vi "IIR Filter for N Chan-modified.vi"(4 "optional IIR filter specifications":T2={"Lower PB"=100.0, "Upper PB"=0.0, "Lower SB"=200.0, "Upper SB"=0.0, "PB Gain"=0.0, "SB Gain"=-60.0, "Scale"=TRUE} {"PB Gain" format="%0.2f"; "SB Gain" format="%0.2f"; "Lower SB" format="%0.2p"; "Upper SB" format="%0.2f"; "Lower PB" format="%0.2p"; "Upper PB" format="%0.2f"}, 6 "IIR filter specifications":T3={"Topology"=enum."Butterworth", "Type"=enum."Lowpass", "Order"=1, "Lower Fc"=100.0, "Upper Fc"=200.0, "PB Ripple"=1.0, "SB Attenuation"=60.0} {"PB Ripple" format="%0.2f"; "Lower Fc" format="%0.2p"; "SB Attenuation" format="%0.2f"; "Upper Fc" format="%0.2p"}, 7 "reset filters":bool, 8 "error in (no error)":errorcluster, 11 "signal(s) in":waveform(dbl)[](array[waveform])) -> (0 "error out":errorcluster, 2 "filter information":T1 {"phase H(w)"."df" format="%.2p"; "phase H(w)"."f0" format="%.2p"; "phase H(w)"."Phase H(w)" format="%.2p"; "magnitude H(w)"."df" format="%.2p"; "magnitude H(w)"."f0" format="%.2p"; "magnitude H(w)"."Mag H(w)" format="%.2p"}, 3 "signal(s) out":waveform(dbl)[](array[waveform]))   [LabVIEW 2015]
doc: "Filters signals in either single or multiple waveforms. If you are filtering multiple waveforms, the VI maintains separate filter states for each waveform. The data types you wire to the <B>signal in</B> and <B>IIR filter specifications</B> inputs determine the polymorphic instance to use."
uses:
  <vilib>/measure/maUtilsandCtls.llb/ma_array_Check Time Signal Continuity.vi
  <vilib>/measure/NI_MAPro.lvlib
  <vilib>/measure/NI_MABase.lvlib
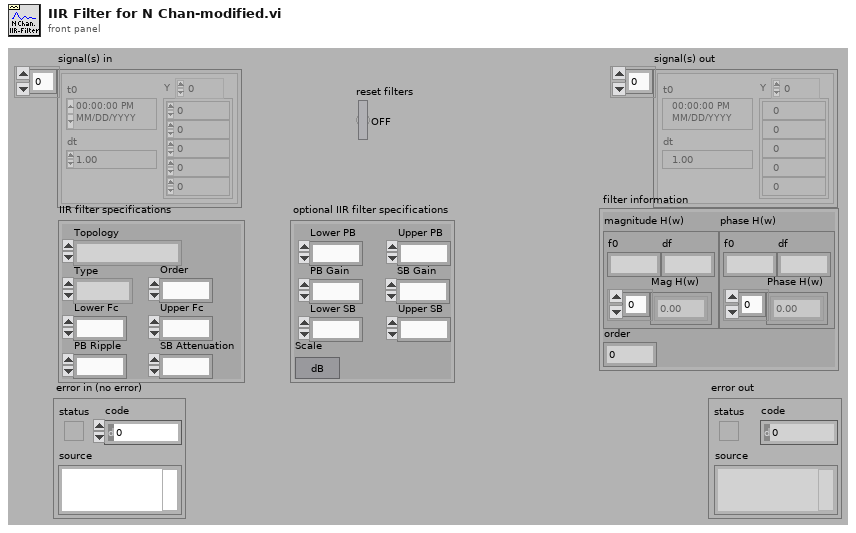
[diagram p1: front panel]
types:
  T1 = cluster{"magnitude H(w)":cluster{"f0":dbl, "df":dbl, "Mag H(w)":dbl[]}, "phase H(w)":cluster{"f0":dbl, "df":dbl, "Phase H(w)":dbl[]}, "order":i32}
  T2 = cluster{"Lower PB":dbl, "Upper PB":dbl, "Lower SB":dbl, "Upper SB":dbl, "PB Gain":dbl, "SB Gain":dbl, "Scale":bool}
  T3 = cluster{"Topology":enum16{"Off", "Butterworth", "Chebyshev", "Inverse Chebyshev", "Elliptic", "Bessel"}, "Type":enum16{"Lowpass", "Highpass", "Bandpass", "Bandstop"}, "Order":i32, "Lower Fc":dbl, "Upper Fc":dbl, "PB Ripple":dbl, "SB Attenuation":dbl}
  T4 = cluster{"filter structure":enum32{"IIR 2nd Order", "IIR 4th Order"}, "Reverse Coefficients":dbl[], "Forward Coefficients":dbl[]}
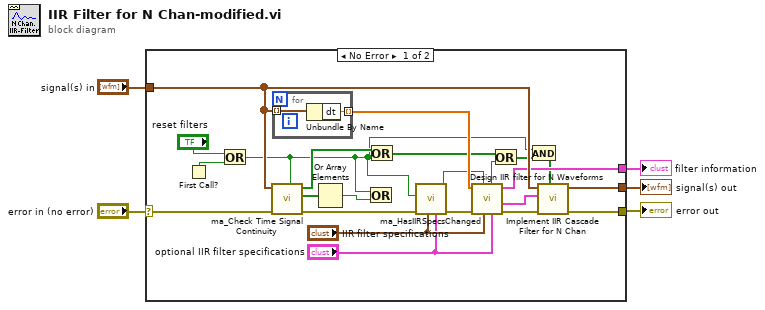
[diagram p0: block diagram]
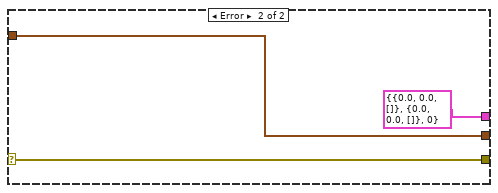
[diagram p2: hidden frame]
diagram:
  n1 = case shown="No Error" "error in (no error)" {
    selector: "error in (no error)" -> [w25 w32]
    tunnel: "signal(s) in" -> [w27 w33]
    tunnel: [w28 w32] -> w4
    tunnel: [w26 w33] -> w3
    tunnel: [w24 T1 {"magnitude H(w)"={"f0"=0.0, "df"=0.0, "Mag H(w)"=[]}, "phase H(w)"={"f0"=0.0, "df"=0.0, "Phase H(w)"=[]}, "order"=0} ("Filter Information")] -> w1
    frame No Error {
      n2 = First Call?() -> (First Call?: T/F=w10:bool)
      n3 = Or(x="reset filters", y=w10) -> (x .or. y?=w6:bool)
      n4 = call-poly <vilib>:"ma_Check Time Signal Continuity.vi"("Ignore input time stamp"=w6, "error in (no error)"=w25, "waveforms"=w27) -> ("error out"=w16:errorcluster, "dt changed"=w20:bool[], "t0 changed"=w13:bool[])  [unwired: 5 in, 1 out]
      n5 = for {
        tunnel: w27 -> [w30] mode=indexing
        tunnel: [w29] -> w21 mode=indexing
        n6 = Unbundle By Name(w30) -> ("dt"=w29:dbl)
      }
      n7 = Or Array Elements(Boolean array=w20) -> (logical OR=w14:bool)
      n8 = Or(x=w6, y=w14) -> ()  [unwired: 1 out]
      n9 = Or(x=w13, y=w6) -> (x .or. y?=w12:bool[])
      n10 = call <vilib>:"ma_HasIIRSpecsChanged.vi"("optional IIR filter specifications"="optional IIR filter specifications", "IIR filter specifications"="IIR filter specifications", "error in (no error)"=w16, "redesign filter"=w6) -> ("error out"=w17:errorcluster, "ValsDifferent?"=w15:bool)  [unwired: 6 in]
      n11 = call <vilib>:"Design IIR filter for N Waveforms.vi"("Optional Filter Specifications"="optional IIR filter specifications", "Filter specifications"="IIR filter specifications", "Reset history"=w15, "error in"=w17, "arrdt"=w21) -> ("error out"=w22:errorcluster, "IIR Filter Cluster"=w23:T4, "Filter Information"=w24:T1, "reset filters"=w19:bool)  [unwired: 3 in]
      n12 = Or(x=w12, y=w19) -> (x .or. y?=w18:bool[])
      n13 = And(x=w6, y=w18) -> (x .and. y?=w7:bool[])
      n14 = call <vilib>:"Implement IIR Cascade Filter for N Chan.vi"("reset filter states"=w7, "error in (no error)"=w22, "IIR Filter Cluster"=w23, "arrWaveforms"=w27) -> ("error out"=w28:errorcluster, "arrFilteredWaveforms"=w26:waveform(dbl)[])  [unwired: 6 in]
    }
    frame Error {
    }
  }
  "error out" <- w4
  "signal(s) out" <- w3
  "filter information" <- w1
